vi "TEST_bench_sat_op_fxp_16_5.vi"(7 "N_sat":i32) -> ()   [LabVIEW 2017]
panel:
  out "S_of_uk_fp":sgl[](array[numeric])
  out "S_of_uk_fxp":fxp<+/-,32,10>[](array[numeric])
  in  "uk":sgl[](array[numeric]) format="%#_13g"
  in  "numIter":i32
  in  "d_s":fxp<+/-,16,5>[](array[numeric])=[0.0, 0.82861328125, 1.8125, 2.8671875, 4.03173828125, 5.2001953125, 7.20166015625]
  in  "satw_s":fxp<+/-,16,5>[](array[numeric])=[0.0, 0.0, 0.0, 0.0, 0.0, 0.0, 0.0]
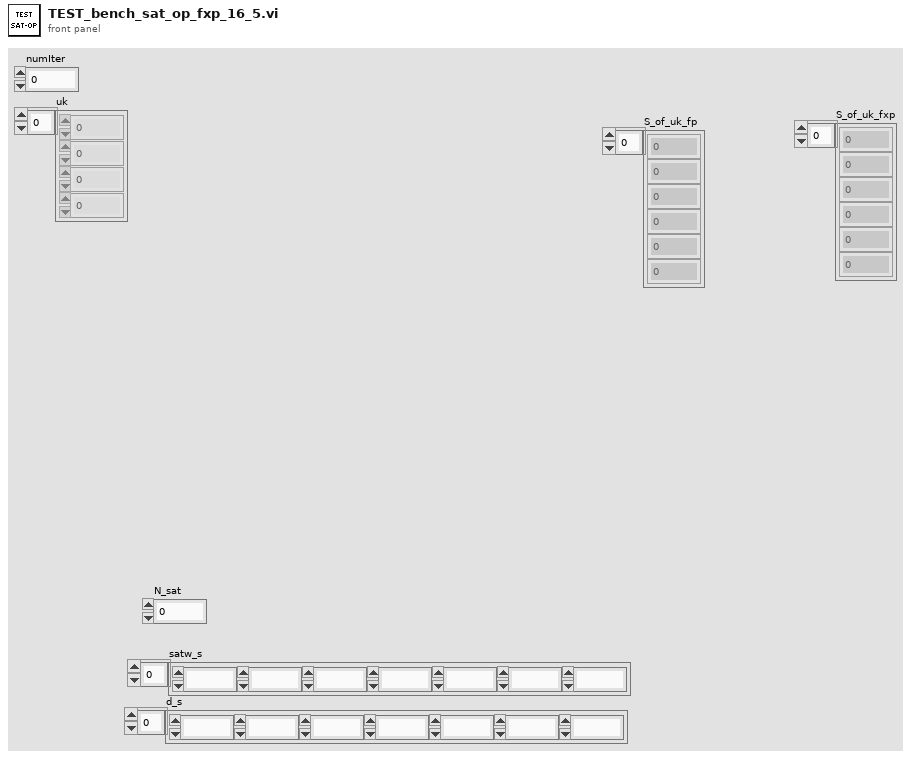
[diagram p1: front panel]
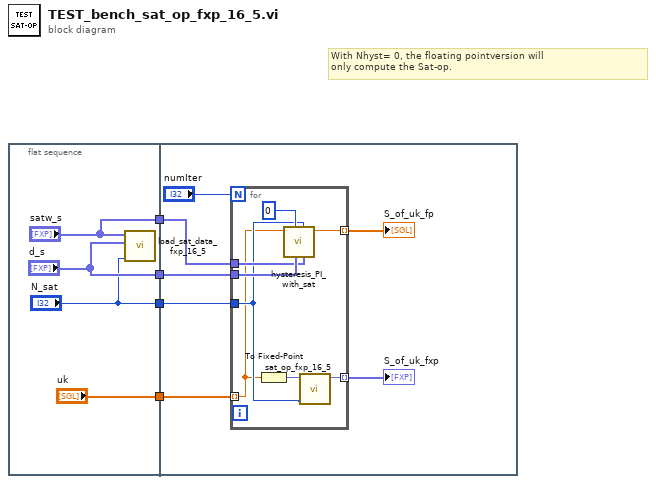
[diagram p0: block diagram]
diagram:
  # "With Nhyst= 0, the floating pointversion will\nonly compute the Sat-op."
  n1 = flat-sequence {
    tunnel: ["uk"] -> w4
    tunnel: ["satw_s"] -> w3
    tunnel: ["d_s"] -> w2
    tunnel: ["N_sat"] -> w1
    tunnel: w4 -> [w12]
    tunnel: w3 -> [w11]
    tunnel: w2 -> [w10]
    tunnel: w1 -> [w9]
    frame #0 {
      n2 = call "load_sat_data_fxp_16_5.vi"("N_sat"="N_sat", "sat_d_s"="d_s", "sat_w_s"="satw_s") -> ()  [unwired: 9 in]
    }
    frame #1 {
      n3 = for {
        N: "numIter" -> [_]
        tunnel: [w18] -> w14 mode=indexing
        tunnel: w11 -> [w20]
        tunnel: w10 -> [w21]
        tunnel: [w22] -> w15 mode=indexing
        tunnel: w12 -> [w16] mode=indexing
        tunnel: w9 -> [w17]
        n4 = To Fixed-Point(number=w16) -> (fixed-point=w19:fxp<+/-,16,5>)  [unwired: 1 in]
        n5 = call "hysteresis_PI_with_sat.vi"("wsat_s"=w20, "N_sat"=w17, "d_s"=w21, "N_hyst"=0, "uk"=w16) -> ("H_of_ik"=w22:sgl)  [unwired: 5 in, 1 out]
        n6 = call "sat_op_fxp_16_5.vi"("N_sat"=w17, "uk_in"=w19) -> ("Hinv(uk)"=w18:fxp<+/-,32,10>)  [unwired: 9 in]
      }
      "S_of_uk_fxp" <- w14
      "S_of_uk_fp" <- w15
    }
  }
